vi "Include_in_Preview.vi"(8 "error in (no error)":errorcluster, 11 "AB_Source in":refnum<class "AB_Source.lvclass">) -> (0 "error out":errorcluster, 2 "includeInPreview":bool)   [LabVIEW 2020, in "AB_Source.lvclass"]
uses:
  <vilib>/AppBuilder/AB_Classes/Source/AB_Source.lvclass
  <vilib>/AppBuilder/AB_Classes/Source/AB_Source.lvclass/AB_Source.ctl
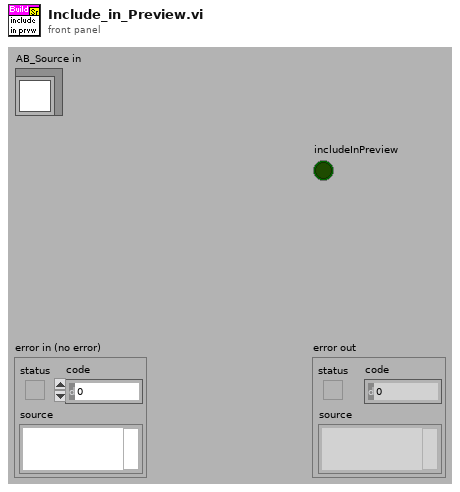
[diagram p1: front panel]
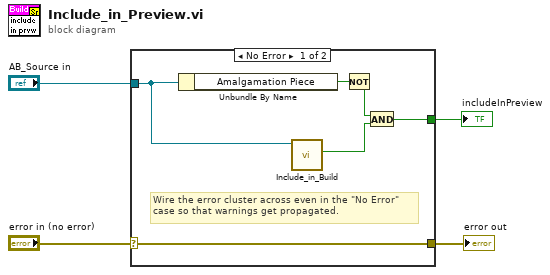
[diagram p0: block diagram]
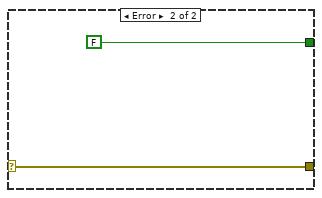
[diagram p2: hidden frame]
diagram:
  n1 = case shown="No Error" "error in (no error)" {
    selector: "error in (no error)" -> [w10 w12]
    tunnel: [w10 w12] -> w3
    tunnel: "AB_Source in" -> [w9 _]
    tunnel: [w5 FALSE] -> w1
    frame No Error {
      # "Wire the error cluster across even in the \"No Error\"\ncase so that warnings get propagated."
      n2 = Unbundle By Name(w9) -> ("Amalgamation Piece"=w7:bool)
      n3 = call-dynamic "Include_in_Build.vi"("AB_Source in"=w9) -> ("includeInBuild"=w8:bool)  [unwired: 8 in, 2 out]
      n4 = Not(x=w7) -> (.not. x?=w6:bool)
      n5 = And(x=w6, y=w8) -> (x .and. y?=w5:bool)
    }
    frame Error {
    }
  }
  "error out" <- w3
  "includeInPreview" <- w1
